vi "configuration methods.vi"() -> (0 "error out":errorcluster, 2 "modules equal":bool, 3 "channels equal":bool)   [LabVIEW 2013, in "Shared Memory Tests.lvlib"]
doc: "Copyright 2016 National Instruments Corporation\n\nLicensed under the Apache License, Version 2.0 (the \"License\"); you may not use this file except in compliance with the License. You may obtain a copy of the License at http://www.apache.org/licenses/LICENSE-2.0\nUnless required by applicable law or agreed to in writing, software distributed under the License is distributed on an \"AS IS\" BASIS, WITHOUT WARRANTIES OR CONDITIONS OF ANY KIND, either express or implied. See the License for the specific language governing permissions and limitations under the License."
uses:
  Shared Memory Tests.lvlib
  module/configuration/Shared Memory Configuration.lvclass
panel:
  out "created channels":i32
  out "configuration channels":i32
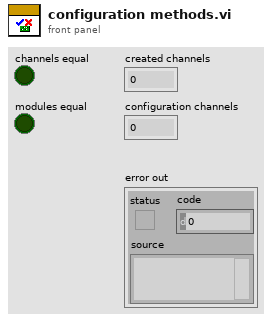
[diagram p1: front panel]
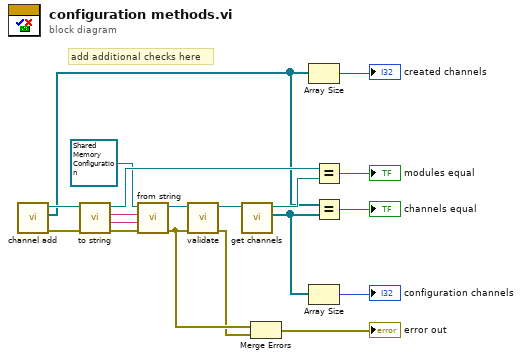
[diagram p0: block diagram]
diagram:
  # "add additional checks here"
  n1 = call "channel add.vi"() -> ("error out"=w12:errorcluster, "channels"=w7:refnum<class "TBM channel.lvclass">[], "configuration out"=w13:refnum<class "Shared Memory Configuration.lvclass">)  [unwired: 7 in, 2 out]
  n2 = call-dynamic "to string.vi"("error in"=w12, "shared memory module configuration"=w13) -> ("error out"=w19:errorcluster, "data"=w18:string, "version"=w17:string, "shared memory module configuration out"=w9:refnum<class "Shared Memory Configuration.lvclass">)  [unwired: 6 in]
  n3 = call-dynamic "from string.vi"("error in"=w19, "data"=w18, "version"=w17, "shared memory module configuration"=refnum<class "Shared Memory Configuration.lvclass"> refnum ("tag bus configurable plugin module configuration")) -> ("error out"=w3:errorcluster, "shared memory module configuration out"=w16:refnum<class "Shared Memory Configuration.lvclass">)  [unwired: 6 in]
  n4 = call-dynamic "validate.vi"("error in"=w3, "shared memory module configuration"=w16) -> ("error out"=w2:errorcluster, "shared memory module configuration out"=w14:refnum<class "Shared Memory Configuration.lvclass">)  [unwired: 8 in]
  n5 = call-dynamic "get channels.vi"("shared memory module configuration"=w14) -> ("channels"=w6:refnum<class "TBM channel.lvclass">[], "shared memory module configuration out"=w10:refnum<class "Shared Memory Configuration.lvclass">)  [unwired: 9 in]
  n6 = Merge Errors(w3, w2) -> (→"error out":errorcluster)
  n7 = Array Size(array=w7) -> (size(s)=→"created channels":i32)
  n8 = Array Size(array=w6) -> (size(s)=→"configuration channels":i32)
  n9 = Equal?(x=w9, y=w10) -> (x = y?=→"modules equal":bool)
  n10 = Equal?(x=w7, y=w6) -> (x = y?=→"channels equal":bool)
